vi "Bands to value.vi"(3 "Multiplier":T1, 4 "Digit 2":T2, 5 "Digit":T2) -> (1 "vn":dbl)   [LabVIEW 2018]
uses:
  Digit--control.ctl
  Multiplier--control.ctl
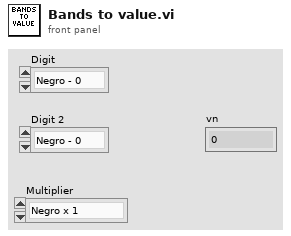
[diagram p1: front panel]
types:
  T1 = typedef "Multiplier--control.ctl" = enum16{"Negro x 1", "Marron x 10", "Rojo x 100", "Naranja x 1K", "Amarillo x 10K", "Verde x 100K", " Azul x 1M", "Violeta x 10M ", "Oro x 0.1", "Plata x 0.01"}
  T2 = typedef "Digit--control.ctl" = enum16{"Negro - 0", "Marron - 1", "Rojo - 2", "Naranja - 3", "Amarillo - 4", "Verde - 5", "Azul - 6", "Violeta - 7", "Gris - 8", "Blanco - 9"}
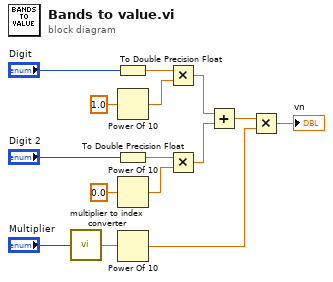
[diagram p0: block diagram]
diagram:
  n1 = call "multiplier to index converter.vi"("Multiplier"="Multiplier") -> ("Index"=w8:dbl)  [unwired: 4 in]
  n2 = To Double Precision Float(number="Digit") -> (double precision float=w2:dbl)
  n3 = Power Of 10(x=1.0) -> (10^x=w15:dbl)
  n4 = To Double Precision Float(number="Digit 2") -> (double precision float=w1:dbl)
  n5 = Power Of 10(x=0.0) -> (10^x=w11:dbl)
  n6 = Power Of 10(x=w8) -> (10^x=w5:dbl)
  n7 = Multiply(x=w2, y=w15) -> (x*y=w7:dbl)
  n8 = Multiply(x=w1, y=w11) -> (x*y=w6:dbl)
  n9 = Add(x=w7, y=w6) -> (x+y=w4:dbl)
  n10 = Multiply(x=w4, y=w5) -> (x*y=→"vn":dbl)
